vi "Create Framework Performance.vi"(8 "error in (no error)":errorcluster) -> (0 "error out":errorcluster, 3 "Framework Performance":refnum<class "Framework Performance.lvclass">)   [LabVIEW 2017, in "Data Sharing Framework Engine.lvlib" / "Framework Performance.lvclass"]
uses:
  Framework Performance.lvclass
  <vilib>/National Instruments/Memory Manager/Classes/Pointer/Memory.Pointer.lvclass/Memory.Pointer.ctl
  Framework Performance.lvclass/Framework Performance.ctl
  <vilib>/National Instruments/Memory Manager/Classes/Pointer/Memory.Pointer.New.4B.vi
  <vilib>/National Instruments/Memory Manager/Classes/Pointer/Memory.Pointer.Allocate.vi
  <vilib>/National Instruments/Memory Manager/Classes/Pointer/Memory.Pointer.Get Size.vi
  <vilib>/National Instruments/Memory Manager/Classes/Pointer/Memory.Pointer.Copy All.vi
  <vilib>/National Instruments/Memory Manager/Classes/Pointer/Memory.Pointer.Set Address.vi
  <vilib>/National Instruments/Memory Manager/Classes/Pointer/Memory.Pointer.Set Size.vi
  <vilib>/National Instruments/Memory Manager/Classes/Pointer/Memory.Pointer.Set Allocated.vi
  <vilib>/National Instruments/Memory Manager/Classes/Pointer/Memory.Pointer.Copy.vi
  <vilib>/National Instruments/Memory Manager/Classes/Pointer/Memory.Pointer.Copy.No Check.vi
  <vilib>/National Instruments/Memory Manager/Classes/Pointer/Memory.Pointer.Parameter Check.Subset.vi
  <vilib>/National Instruments/Memory Manager/Classes/Pointer/Memory.Pointer.Parameter Check.Null Pointer.vi
  <vilib>/National Instruments/Memory Manager/Classes/Pointer/Memory.Pointer.Get Address.vi
  <vilib>/National Instruments/Memory Manager/Classes/Pointer/Memory.Pointer.Errors.vi
  <vilib>/National Instruments/Memory Manager/Classes/Pointer/Memory.Pointer.Errors.Out of Bounds.vi
  <vilib>/National Instruments/Memory Manager/Classes/Pointer/Memory.Pointer.Errors.Null Pointer.vi
  <vilib>/NI/Static Error Handling/VIs/Static Error Handling.Source Buffer.Write.String.vi
  <vilib>/National Instruments/Memory Manager/Classes/Pointer/Memory.Pointer.Errors.Write Pointer Size.vi
  <vilib>/National Instruments/Memory Manager/Classes/Pointer/Memory.Pointer.Errors.Create Error.vi
  <vilib>/NI/Static Error Handling/VIs/Static Error Handling.Source Buffer.Write.Numeric.Scalar.Base10.vi
  <vilib>/NI/Static Error Handling/VIs/Static Error Handling.Source Buffer.Write.Numeric.Scalar.Base10 (U64).vi
  <vilib>/NI/Static Error Handling/VIs/Static Error Handling.Error Cluster Constant.vi
  <vilib>/NI/Static Error Handling/VIs/Static Error Handling.Error Cluster Constant (512B).vi
  <vilib>/NI/Static Error Handling/VIs/Static Error Handling.Parameters.Status.Set.vi
  <vilib>/NI/Static Error Handling/VIs/Static Error Handling.Parameters.Code.Set.vi
  <vilib>/NI/Static Error Handling/VIs/Static Error Handling.Parameters.VI Source.Set.vi
  <vilib>/National Instruments/Memory Manager/Constants/Memory.Constants.vi
  <vilib>/National Instruments/Memory Manager/Constants/Memory.Constants.Library Name.vi
  <vilib>/National Instruments/Memory Manager/Classes/Pointer/Memory.Pointer.Errors.Get Info.vi
  <vilib>/National Instruments/Memory Manager/Classes/Pointer/Memory.Pointer.lvclass
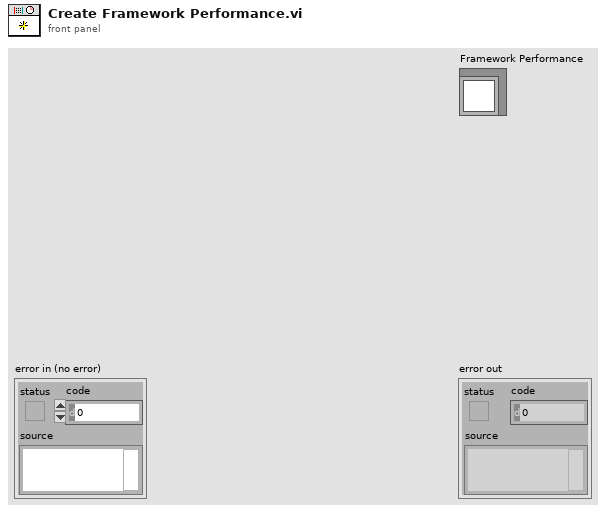
[diagram p1: front panel]
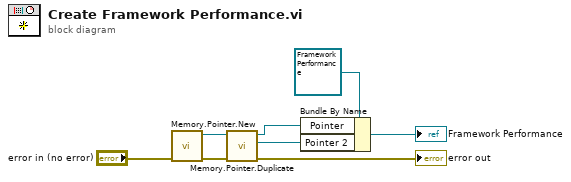
[diagram p0: block diagram]
diagram:
  n1 = call-poly <vilib>:"Memory.Pointer.New.vi"("error in (no error)"="error in (no error)") -> ("error out"=w3:errorcluster, "Pointer"=w6:refnum<class "Memory.Pointer.lvclass">)  [unwired: 9 in]
  n2 = call <vilib>:"Memory.Pointer.Duplicate.vi"("error in (no error)"=w3, "Pointer in"=w6) -> ("error out"=→"error out":errorcluster, "new duplicate Pointer"=w5:refnum<class "Memory.Pointer.lvclass">, "Pointer out"=w4:refnum<class "Memory.Pointer.lvclass">)  [unwired: 7 in]
  n3 = Bundle By Name(cluster=refnum<class "Framework Performance.lvclass"> refnum ("Framework Performance in"), "Pointer"=w4, "Pointer 2"=w5) -> (→"Framework Performance":refnum<class "Framework Performance.lvclass">)
